vi "TablaMultiplicar.vi"() -> ()   [LabVIEW 2020]
panel:
  in  "Renglones":i32
  in  "Columnas":i32
  out "Array":i32[][](array[numeric])
  out "Resultado":i32
  in  "Segundo numero":i32
  in  "Primer numero":i32
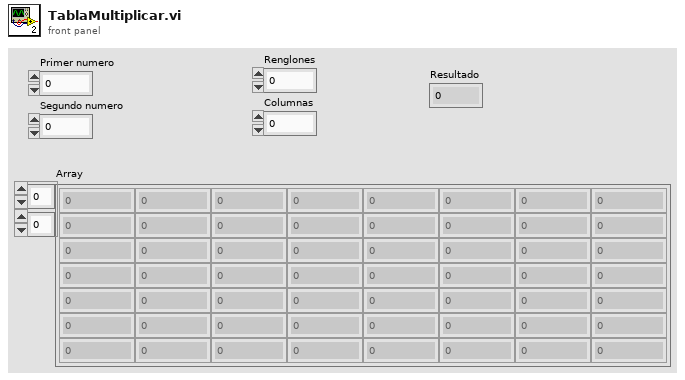
[diagram p1: front panel]
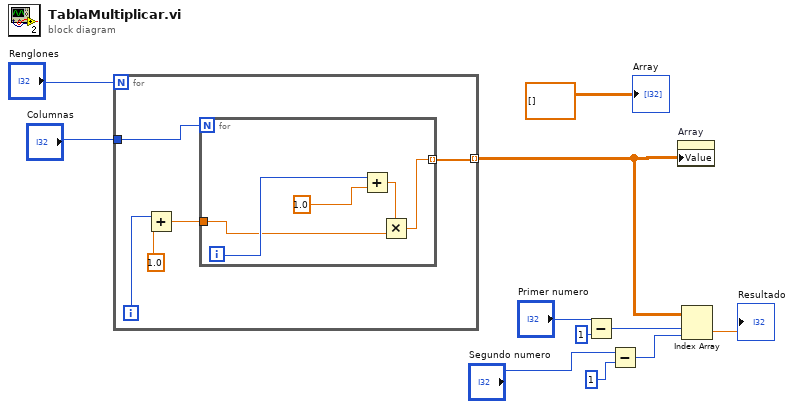
[diagram p0: block diagram]
diagram:
  n1 = for {
    N: "Renglones" -> [_]
    tunnel: "Columnas" -> [w16]
    tunnel: [w12] -> w10 mode=indexing
    i -> [w14]
    n2 = Add(x=w14, y=1.0) -> (x+y=w13:dbl)
    n3 = for {
      N: w16 -> [_]
      tunnel: w13 -> [w19]
      tunnel: [w18] -> w12 mode=indexing
      i -> [w20]
      n4 = Add(x=w20, y=1.0) -> (x+y=w17:dbl)
      n5 = Multiply(x=w17, y=w19) -> (x*y=w18:dbl)
    }
  }
  n6 = Subtract(x="Primer numero", y=1) -> (x-y=w6:i32)
  n7 = Subtract(x="Segundo numero", y=1) -> (x-y=w3:i32)
  n8 = property on="Array" class="Arr (strict)"("Value"=w10) -> ()  [unwired: 2 in, 2 out]
  n9 = Index Array(array=w10, index (row)=w6, index (col)=w3) -> (element=→"Resultado":dbl)
  "Array" <- dbl[][] [] ("Array")
